vi "Module - MQTT Client.vi"(8 "error in (no error)":errorcluster) -> (0 "error in (no error) 2":errorcluster)   [LabVIEW 2020]
uses:
  <vilib>/LabVIEW Open Source Project/MQTT Connection/MQTT_Base/Base Class/MQTT_Base.lvclass
  <vilib>/LabVIEW Open Source Project/MQTT Client/Client class/Client.lvclass
  Control/State - MQTT Client.ctl
  Shared/Control/State - eFGV.ctl
  <vilib>/LabVIEW Open Source Project/MQTT TCP Connection/MQTT_TCP/Connection/TCPConnection.lvclass
  <vilib>/LabVIEW Open Source Project/MQTT Control Packets/Control Packets/CONNACK/Connect Return Code -- enum.ctl
  <vilib>/LabVIEW Open Source Project/MQTT Control Packets/Control Packets/CONNACK/CONNACK.lvclass
  <vilib>/LabVIEW Open Source Project/MQTT Control Packets/Control Packets/PUBLISH/PUBLISH.lvclass
  <vilib>/LabVIEW Open Source Project/MQTT Client/Client class/Public Events -- cluster.ctl
  Control/MQTT Sub Unsub.ctl
  Control/MQTT Connection Settings.ctl
  Control/MQTT Send Data.ctl
  Control/MQTT Received Data.ctl
  <vilib>/LabVIEW Open Source Project/OpenSerializer/Serializer/Serializer.lvclass
  Control/Config File Section List.ctl
  C:/Program Files (x86)/National Instruments/LabVIEW 2020/vi.lib/LabVIEW Open Source Project/MQTT Connection/MQTT_Base/Base Class/MQTT_Base.lvclass
  C:/Program Files (x86)/National Instruments/LabVIEW 2020/vi.lib/LabVIEW Open Source Project/MQTT Client/Client class/Client.lvclass
  C:/Program Files (x86)/National Instruments/LabVIEW 2020/vi.lib/LabVIEW Open Source Project/MQTT Connection/MQTT_Connection/Connection/Connection.lvclass
  C:/Program Files (x86)/National Instruments/LabVIEW 2020/vi.lib/LabVIEW Open Source Project/MQTT TCP Connection/MQTT_TCP/Connection/TCPConnection.lvclass
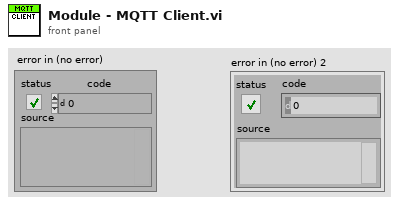
[diagram p1: front panel]
types:
  T1 = cluster{"MQTT Event":refnum<event-registration>, "eFGV Event":refnum<event-registration>}
  T2 = typedef "MQTT Send Data.ctl" = cluster{"Sender Module":string, "Receiving Module":string, "Topic":string, "Data":variant}
  T3 = typedef "MQTT Sub Unsub.ctl" = cluster{"Operation":enum16{"Subscribe", "Unsubscribe"}, "Topic Name":string[]}
  T4 = typedef "MQTT Received Data.ctl" = cluster{"Receiving Module":string, "Topic":string, "Data":variant}
  T5 = typedef "MQTT Connection Settings.ctl" = cluster{"Broker address":string, "Remote port":u16}
  T6 = cluster{"TOut":i32, "User exit":bool, "MQTT Client out":refnum<class "Client.lvclass">, "MQTT Connected":bool, "MQTT Send Data":T2, "MQTT Sub Unsub":T3, "MQTT Received Data":T4, "MQTT Connection Settings":T5, "PUBLISH":refnum<class "PUBLISH.lvclass">}
  T7 = typedef "State - MQTT Client.ctl" = enum16{"Init module", "Register event", "Idle", "Init MQTT Connections", "Init Subscribe Topic", "Create MQTT Client", "Register MQTT Event", "Connect to MQTT Server", "Subscribe MQTT Topic", "Publish to MQTT Tag", "Read MQTT Tag", "Send eFGV", "Check MQTT Connection", "Disconnect from MQTT Server", "Unregister eFGV event", "Close module"}
  T8 = typedef "Config File Section List.ctl" = enum16{"RasPi Setting", "MQTT Server Setting", "MQTT Client Setting", "WiFi Setting", "MQTT Topics"}
  T9 = typedef "State - eFGV.ctl" = enum16{"Init", "Read", "Write", "Close"}
  T10 = typedef "MQTT Client.lvlib/Client.lvclass/Public Events -- cluster.ctl" = cluster{"Connection Status":refnum<user-event>, "Connected":refnum<user-event>, "Application Message":refnum<user-event>}
  T11 = typedef "MQTT Base.lvlib/MQTT_Base.lvclass/Public Events -- cluster.ctl" = cluster{"Stop Event":refnum<user-event>, "Error Event":refnum<user-event>, "Inbound Message":refnum<user-event>}
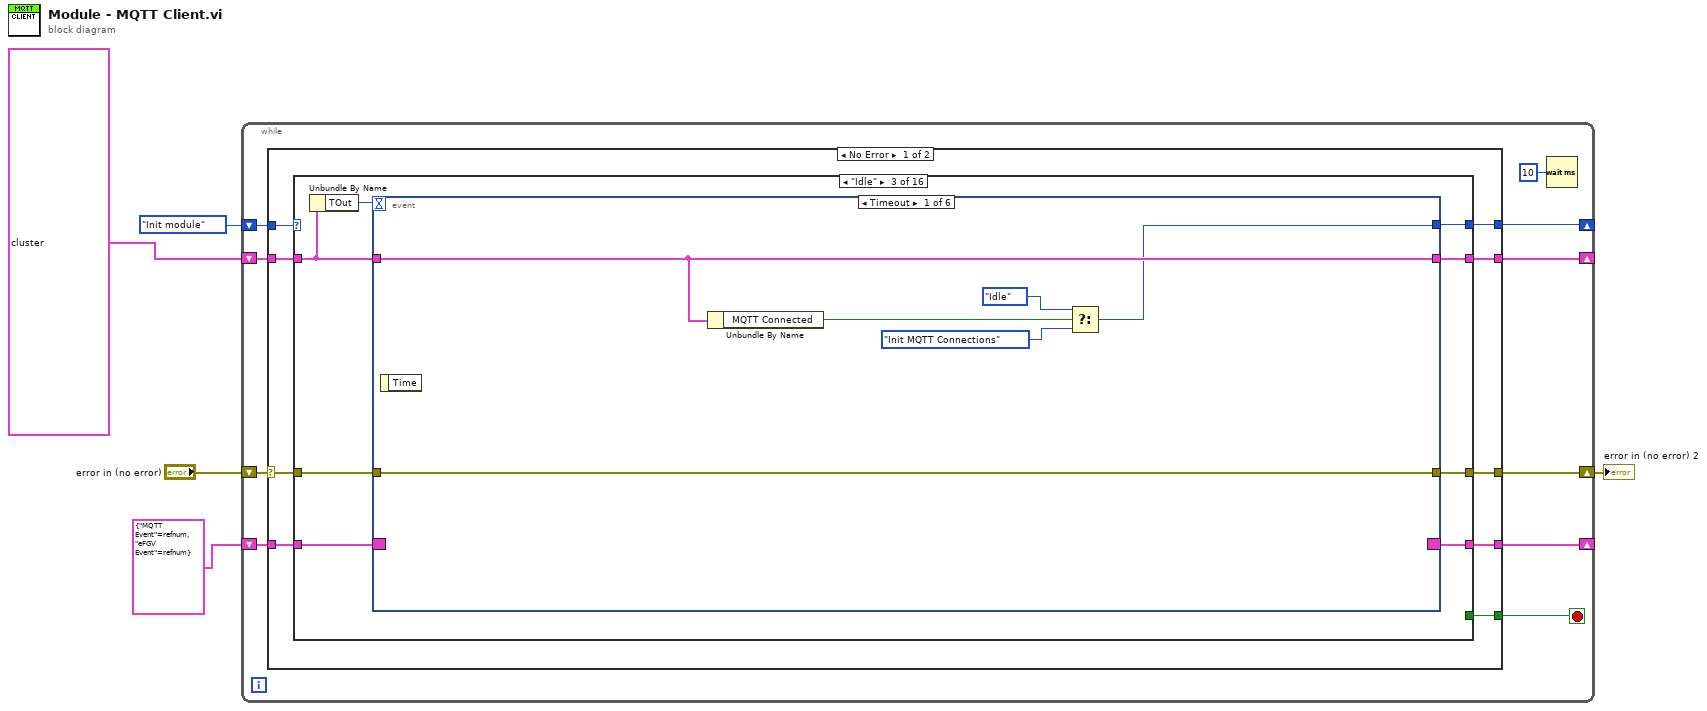
[diagram p0: block diagram]
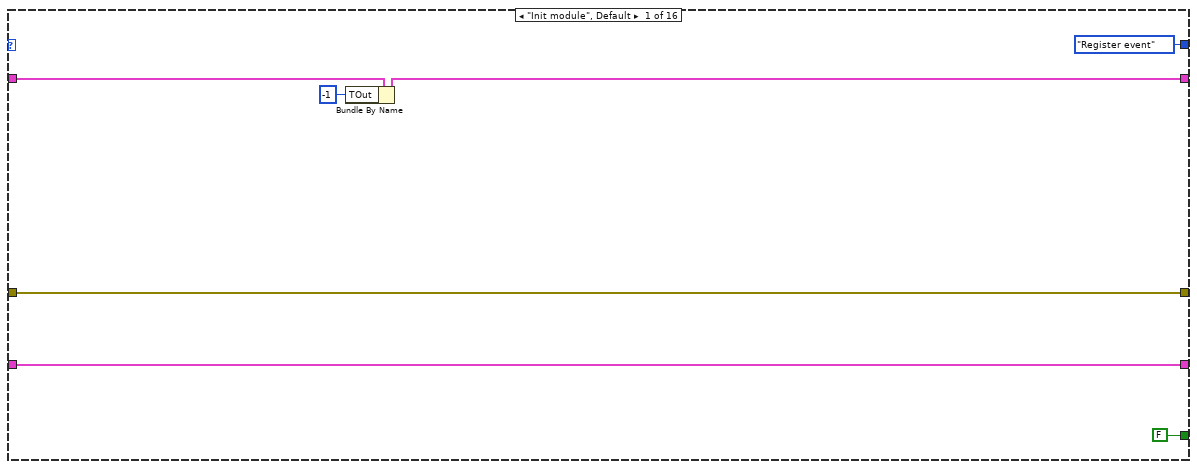
[diagram p2: hidden frame]
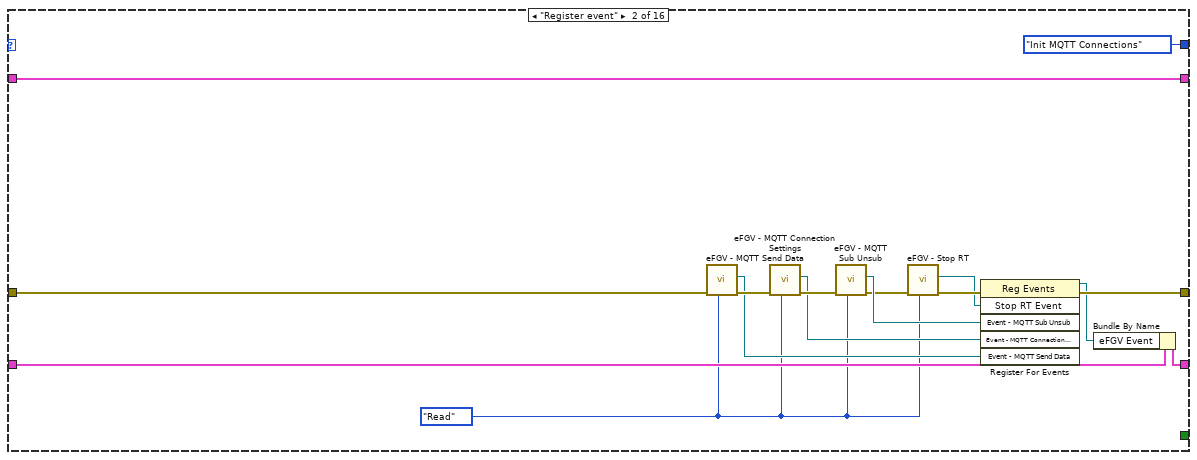
[diagram p3: hidden frame]
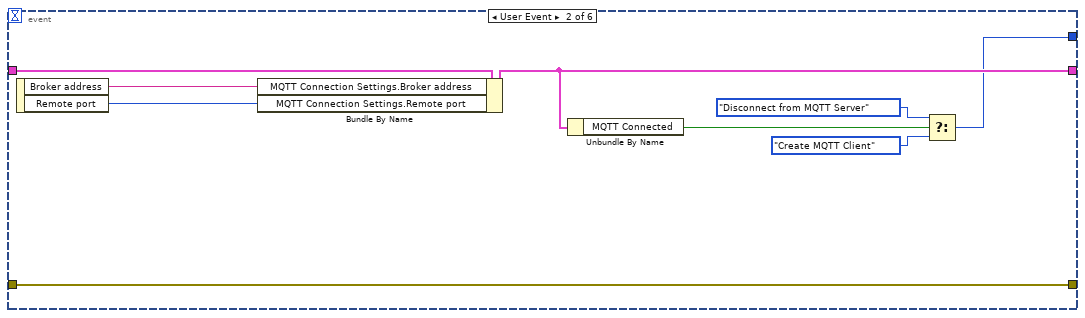
[diagram p4: hidden frame]
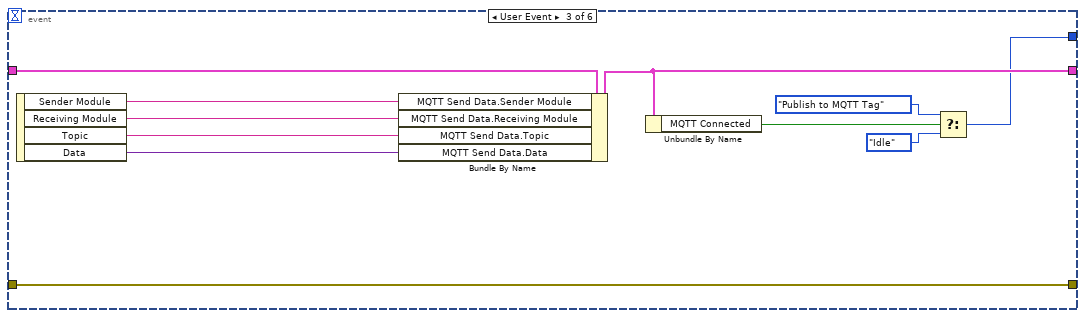
[diagram p5: hidden frame]
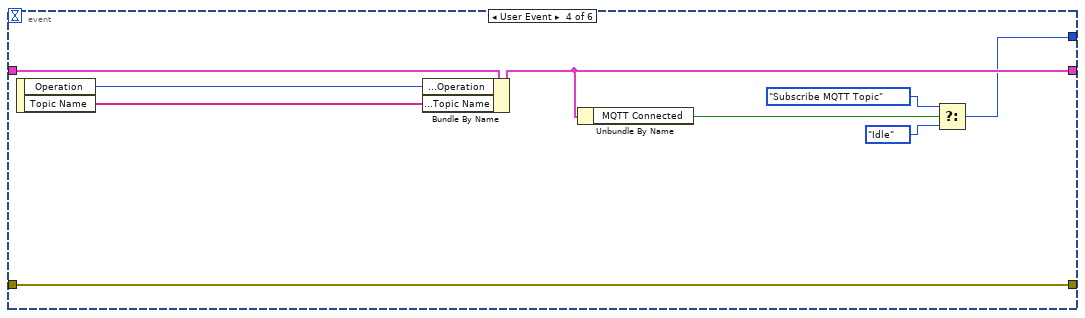
[diagram p6: hidden frame]
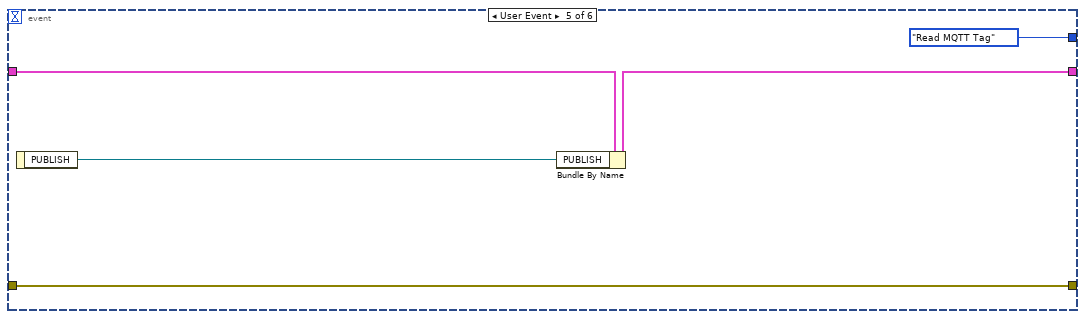
[diagram p7: hidden frame]
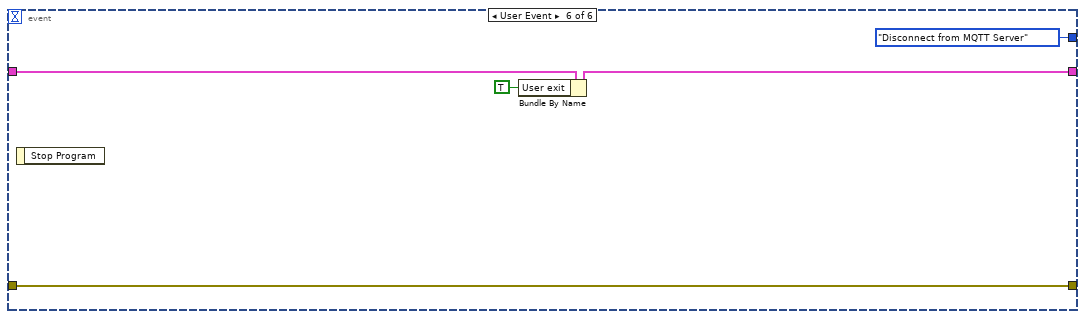
[diagram p8: hidden frame]
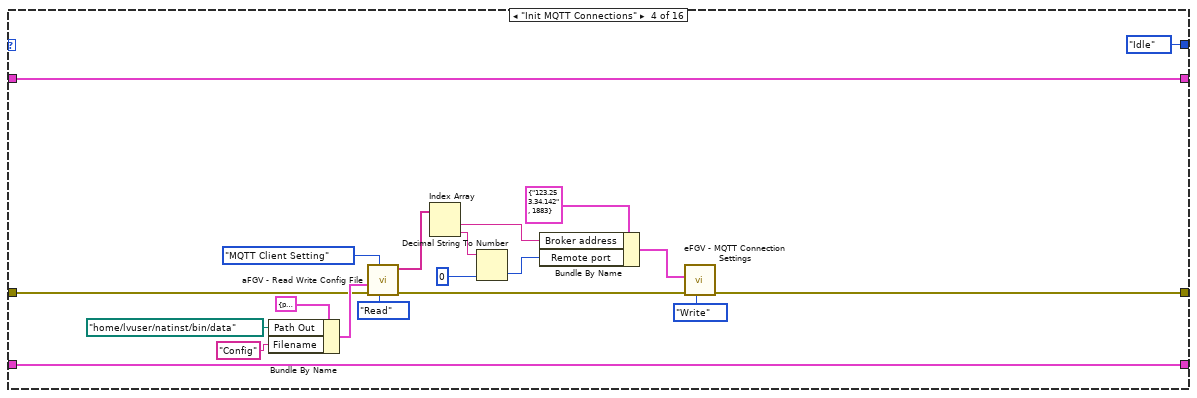
[diagram p9: hidden frame]
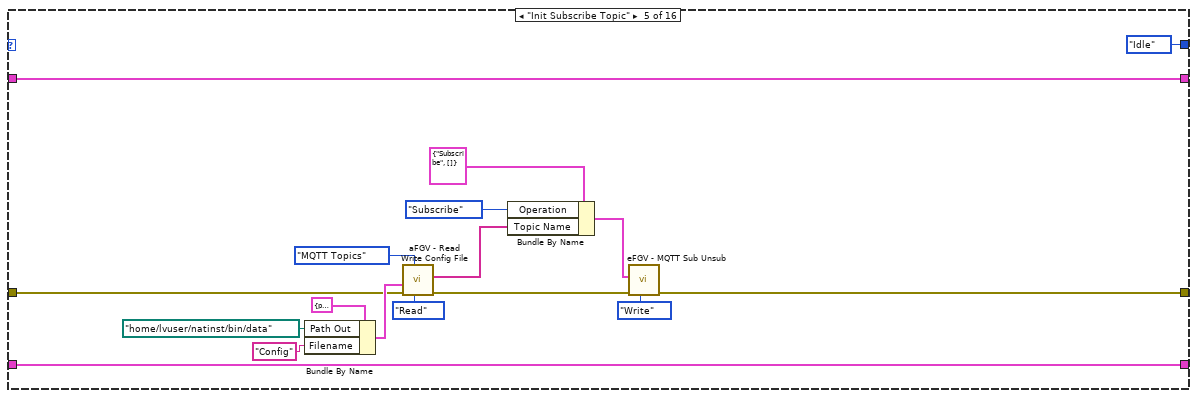
[diagram p10: hidden frame]
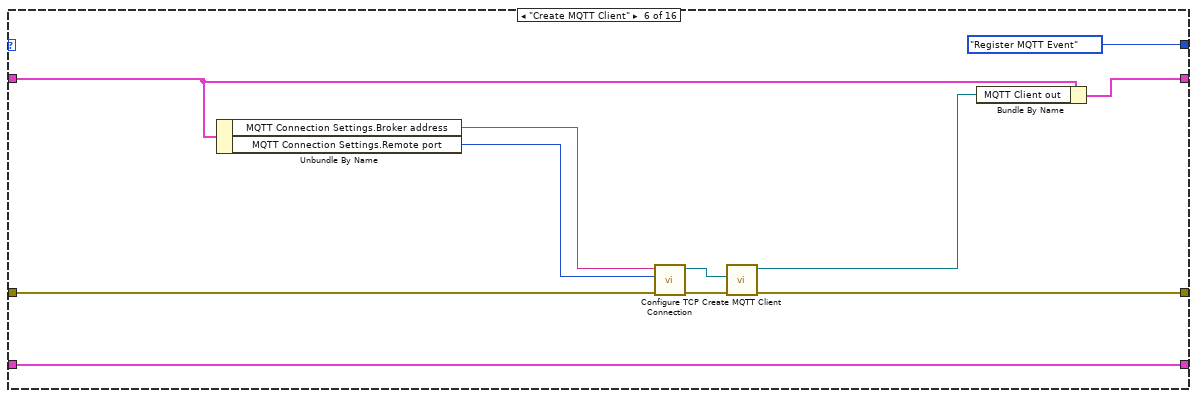
[diagram p11: hidden frame]
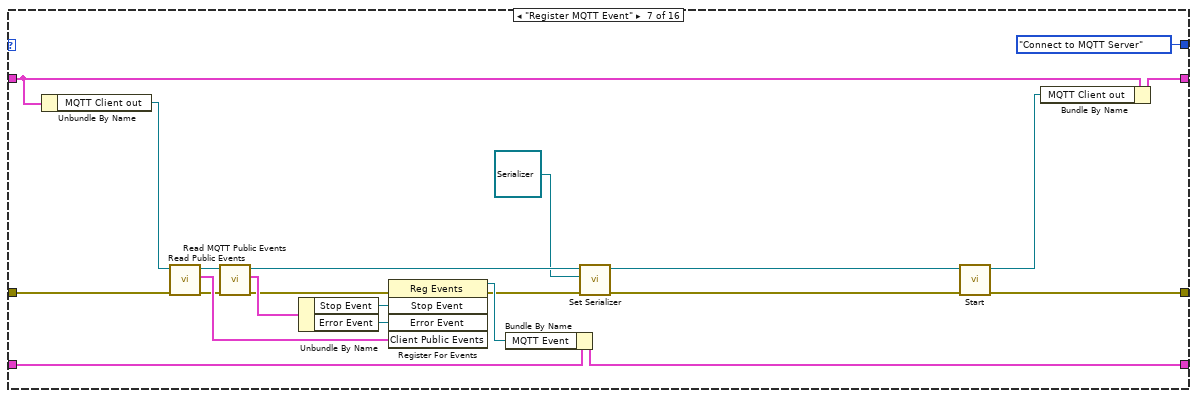
[diagram p12: hidden frame]
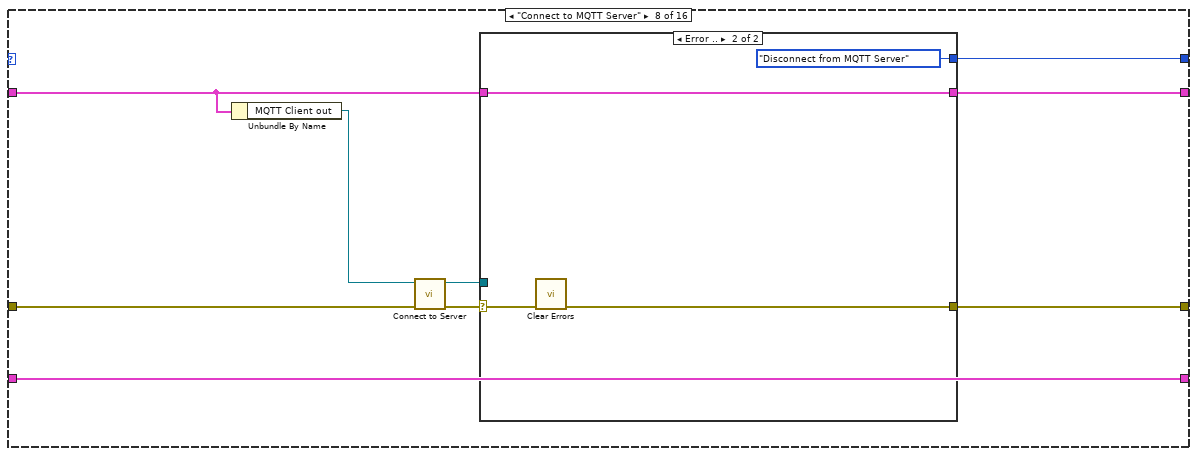
[diagram p13: hidden frame]
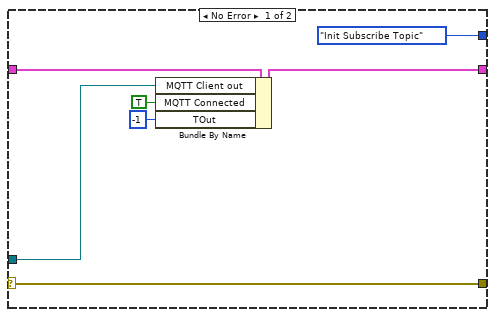
[diagram p14: hidden frame]
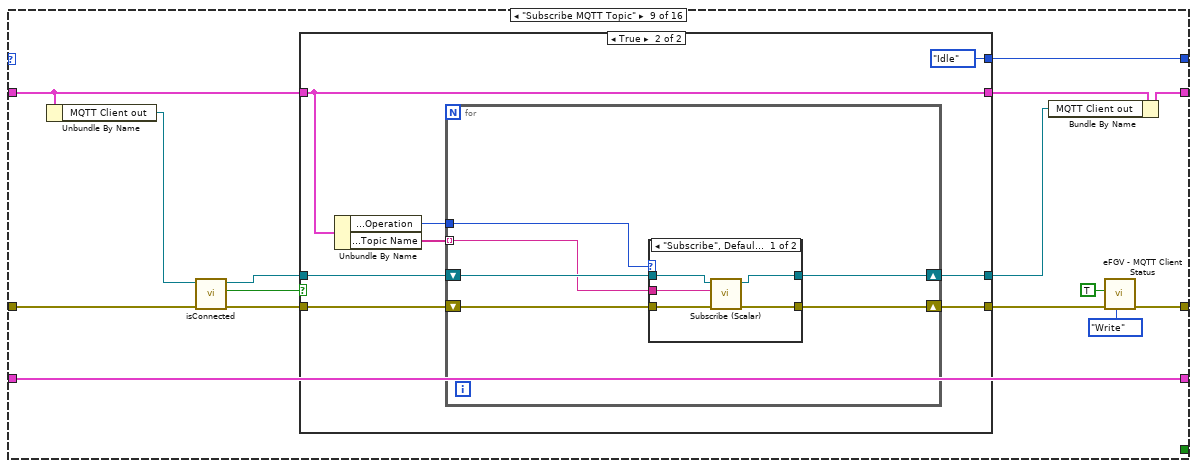
[diagram p15: hidden frame]
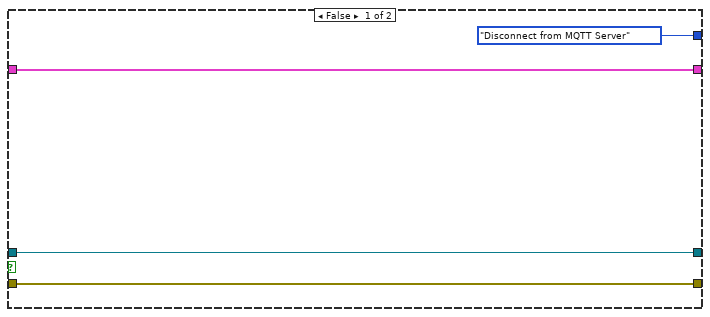
[diagram p16: hidden frame]
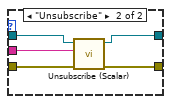
[diagram p17: hidden frame]
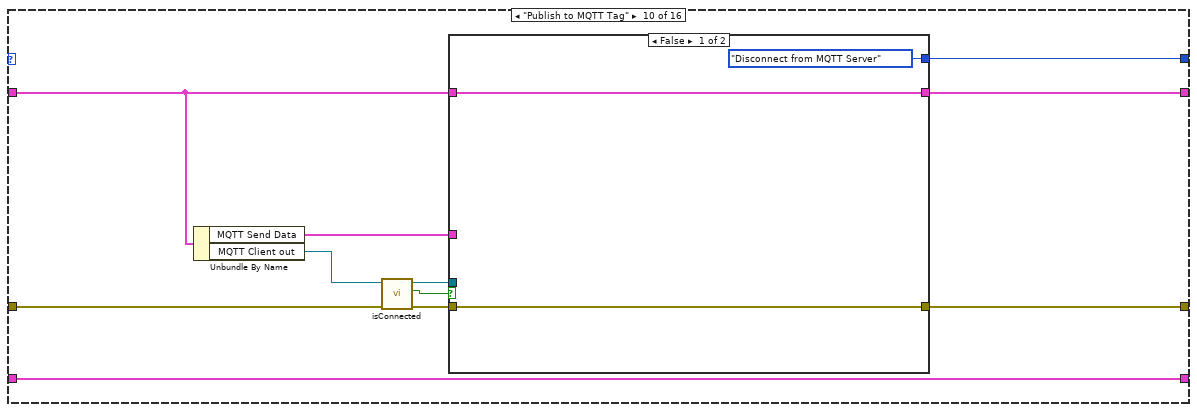
[diagram p18: hidden frame]
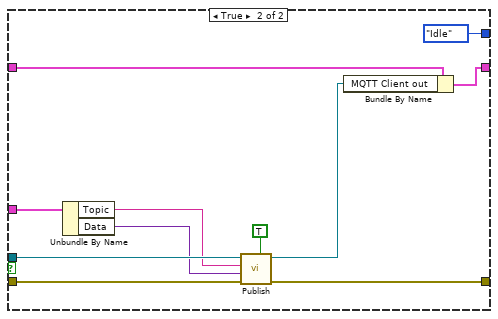
[diagram p19: hidden frame]
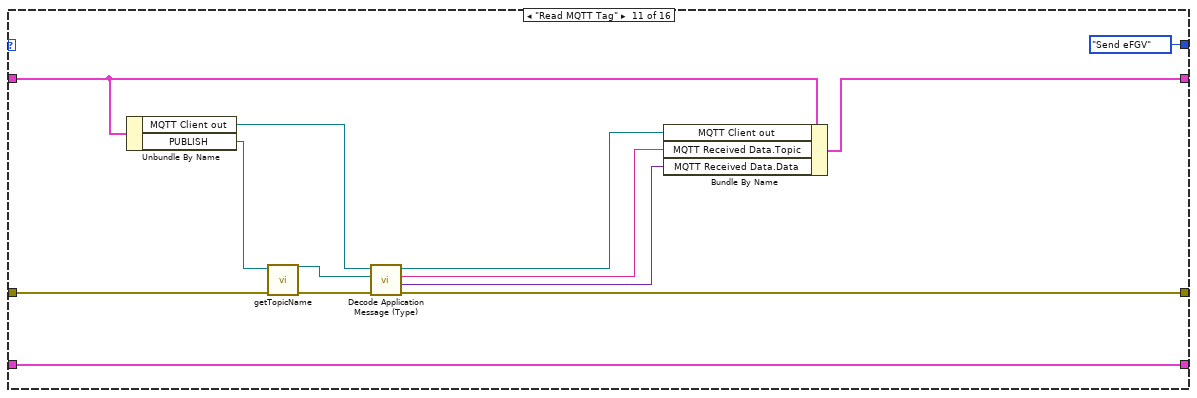
[diagram p20: hidden frame]
diagram:
  n1 = while {
    shift-right: [w12] -> _
    shift-left: State_-_MQTT_Client."Init module" -> [w15]
    shift-right: [w13] -> w1
    shift-left: "error in (no error)" -> [w14]
    shift-right: [w9] -> _
    shift-left: T6 {"TOut"=-1, "User exit"=FALSE, "MQTT Client out"=refnum, "MQTT Connected"=FALSE, "MQTT Send Data"={"Sender Module"="", "Receiving Module"="", "Topic"="", "Data"=variant}, "MQTT Sub Unsub"={"Operation"=enum."Subscribe", "Topic Name"=[]}, "MQTT Received Data"={"Receiving Module"="", "Topic"="", "Data"=variant}, "MQTT Connection Settings"={"Broker address"="123.253.34.142", "Remote port"=1883}, "PUBLISH"=refnum} -> [w10]
    shift-right: [w7] -> _
    shift-left: T1 {"MQTT Event"=refnum, "eFGV Event"=refnum} -> [w8]
    stop <- w11 stop-if-true
    n2 = case shown="No Error" w14 {
      selector: w14 -> [w23 w335]
      tunnel: w15 -> [w24 _]
      tunnel: [w22 w333] -> w13
      tunnel: [w21 State_-_MQTT_Client."Idle"] -> w12
      tunnel: [w20 _] -> w11
      tunnel: w10 -> [w19 w331]
      tunnel: [w18 w331] -> w9
      tunnel: w8 -> [w17 w330]
      tunnel: [w16 w330] -> w7
      frame No Error {
        n3 = case shown="\"Idle\"" w24 {
          tunnel: w23 -> [w31 w38 w49 w107 w125 w145 w162 w178 w204 w242 w265 w277 w284 w302 w321 w329]
          tunnel: [w31 w45 w48 w118 w135 w143 w161 w172 w191 w243 w264 w276 w283 w287 w320 w329] -> w22
          tunnel: [State_-_MQTT_Client."Register event" State_-_MQTT_Client."Init MQTT Connections" w52 State_-_MQTT_Client."Idle" State_-_MQTT_Client."Idle" State_-_MQTT_Client."Register MQTT Event" State_-_MQTT_Client."Connect to MQTT Server" w171 w195 w234 State_-_MQTT_Client."Send eFGV" State_-_MQTT_Client."Idle" _ w293 State_-_MQTT_Client."Close module" State_-_MQTT_Client."Close module"] -> w21
          tunnel: [FALSE _ _ _ _ _ _ _ _ _ _ _ _ _ _ TRUE] -> w20
          tunnel: w19 -> [w28 w47 w51 w120 w137 w140 w158 w177 w200 w236 w262 w278 w282 w295 w324 w328]
          tunnel: [w26 w47 w50 w120 w137 w141 w160 w175 w197 w235 w263 w278 w282 w292 w324 w328] -> w18
          tunnel: w17 -> [w27 w44 w55 w119 w136 w148 w170 w179 w205 w244 w271 w280 w285 w299 w322 w327]
          tunnel: [w27 w43 w54 w119 w136 w148 w156 w179 w205 w244 w271 w280 w285 w298 w322 w327] -> w16
          frame "Init module", Default {
            n4 = Bundle By Name(cluster=w28, "TOut"=-1) -> (w26:T6)
          }
          frame "Register event" {
            w32 = State_-_eFGV."Read" ("State")
            n5 = call "eFGV - MQTT Send Data.vi"("State"=w32, "error in (no error)"=w38) -> ("error out"=w37:errorcluster, "Event - MQTT Send Data"=w36:refnum<user-event>)  [unwired: 8 in]
            n6 = call "eFGV - MQTT Connection Settings.vi"("State"=w32, "error in (no error)"=w37) -> ("error out"=w40:errorcluster, "Event - MQTT Connection Settings"=w39:refnum<user-event>)  [unwired: 8 in]
            n7 = call "eFGV - MQTT Sub Unsub.vi"("State"=w32, "error in (no error)"=w40) -> ("error out"=w35:errorcluster, "Event - MQTT Sub Unsub"=w42:refnum<user-event>)  [unwired: 8 in]
            n8 = call "eFGV - Stop RT.vi"("State"=w32, "error in (no error)"=w35) -> ("error out"=w34:errorcluster, "Stop RT Event"=w33:refnum<user-event>)  [unwired: 8 in]
            n9 = register-events(error in=w34, w33, w42, w39, w36) -> (reference out=w41:refnum<event-registration>, error out=w45:errorcluster)  [unwired: 1 in]
            n10 = Bundle By Name(cluster=w44, "eFGV Event"=w41) -> (w43:T1)
          }
          frame "Idle" {
            n11 = Unbundle By Name(w51) -> ("TOut"=w53:i32)
            n12 = event shown="[0] Timeout" {
              selector: w55 -> [_ _ _ _ _ _]
              dyn-events: [_ _ _ _ _ _] -> w54
              timeout: w53 -> [_ _ _ _ _ _]
              tunnel: [w56 w62 w73 w82 State_-_MQTT_Client."Read MQTT Tag" State_-_MQTT_Client."Disconnect from MQTT Server"] -> w52
              tunnel: w51 -> [w60 w70 w81 w90 w94 w99]
              tunnel: [w60 w63 w74 w86 w93 w98] -> w50
              tunnel: w49 -> [w61 w67 w78 w89 w95 w96]
              tunnel: [w61 w67 w78 w89 w95 w96] -> w48
              event Timeout {
                n13 = event-data() -> ()  [unwired: 1 in, 1 out]
                n14 = Unbundle By Name(w60) -> ("MQTT Connected"=w59:bool)
                n15 = Select(t=State_-_MQTT_Client."Idle", s=w59, f=State_-_MQTT_Client."Init MQTT Connections") -> (s? t:f=w56:T7)
              }
              event User Event {
                n16 = event-data() -> ("Broker address"=w69:string, "Remote port"=w68:u16)  [unwired: 1 in]
                n17 = Bundle By Name(cluster=w70, "MQTT Connection Settings.Broker address"=w69, "MQTT Connection Settings.Remote port"=w68) -> (w63:T6)
                n18 = Unbundle By Name(w63) -> ("MQTT Connected"=w66:bool)
                n19 = Select(t=State_-_MQTT_Client."Disconnect from MQTT Server", s=w66, f=State_-_MQTT_Client."Create MQTT Client") -> (s? t:f=w62:T7)
              }
              event User Event {
                n20 = event-data() -> ("Sender Module"=w72:string, "Receiving Module"=w71:string, "Topic"=w79:string, "Data"=w80:variant)  [unwired: 1 in]
                n21 = Bundle By Name(cluster=w81, "MQTT Send Data.Sender Module"=w72, "MQTT Send Data.Receiving Module"=w71, "MQTT Send Data.Topic"=w79, "MQTT Send Data.Data"=w80) -> (w74:T6)
                n22 = Unbundle By Name(w74) -> ("MQTT Connected"=w77:bool)
                n23 = Select(t=State_-_MQTT_Client."Publish to MQTT Tag", s=w77, f=State_-_MQTT_Client."Idle") -> (s? t:f=w73:T7)
              }
              event User Event {
                n24 = event-data() -> ("Operation"=w87:enum16{"Subscribe", "Unsubscribe"}, "Topic Name"=w88:string[])  [unwired: 1 in]
                n25 = Bundle By Name(cluster=w90, "MQTT Sub Unsub.Operation"=w87, "MQTT Sub Unsub.Topic Name"=w88) -> (w86:T6)
                n26 = Unbundle By Name(w86) -> ("MQTT Connected"=w85:bool)
                n27 = Select(t=State_-_MQTT_Client."Subscribe MQTT Topic", s=w85, f=State_-_MQTT_Client."Idle") -> (s? t:f=w82:T7)
              }
              event User Event {
                n28 = event-data() -> ("PUBLISH"=w91:refnum<class "PUBLISH.lvclass">)  [unwired: 1 in]
                n29 = Bundle By Name(cluster=w94, "PUBLISH"=w91) -> (w93:T6)
              }
              event User Event {
                n30 = event-data() -> ()  [unwired: 1 in, 1 out]
                n31 = Bundle By Name(cluster=w99, "User exit"=TRUE) -> (w98:T6)
              }
            }
          }
          frame "Init MQTT Connections" {
            n32 = Bundle By Name(cluster=cluster{"Path Out":path, "Filename":string} {"Path Out"=path "", "Filename"=""} ("Path File"), "Path Out"=path "/home/lvuser/natinst/bin/data", "Filename"="Config") -> (w108:cluster{"Path Out":path, "Filename":string})
            n33 = call "aFGV - Read Write Config File.vi"("State"=enum16{"Read", "Write", "Delete"}."Read", "Section"=Config_File_Section_List."MQTT Client Setting", "Error In"=w107, "Path File"=w108) -> ("Error Out"=w106:errorcluster, "Data out"=w105:string[])  [unwired: 5 in, 1 out]
            n34 = Index Array(array=w105) -> (element #1=w104:string, element #2=w103:string)  [unwired: 2 in]
            n35 = Decimal String To Number(string=w103, default (0L)=u16 0 ("Remote port")) -> (number=w101:u16)  [unwired: 1 in, 1 out]
            n36 = Bundle By Name(cluster=T5 {"Broker address"="123.253.34.142", "Remote port"=1883} ("MQTT Connection Settings"), "Broker address"=w104, "Remote port"=w101) -> (w116:T5)
            n37 = call "eFGV - MQTT Connection Settings.vi"("State"=State_-_eFGV."Write", "error in (no error)"=w106, "MQTT Connection Settings"=w116) -> ("error out"=w118:errorcluster)  [unwired: 7 in, 1 out]
          }
          frame "Init Subscribe Topic" {
            n38 = Bundle By Name(cluster=cluster{"Path Out":path, "Filename":string} {"Path Out"=path "", "Filename"=""} ("Path File"), "Path Out"=path "/home/lvuser/natinst/bin/data", "Filename"="Config") -> (w127:cluster{"Path Out":path, "Filename":string})
            n39 = call "aFGV - Read Write Config File.vi"("State"=enum16{"Read", "Write", "Delete"}."Read", "Section"=Config_File_Section_List."MQTT Topics", "Error In"=w125, "Path File"=w127) -> ("Error Out"=w126:errorcluster, "Key Names Out"=w122:string[])  [unwired: 5 in, 1 out]
            n40 = Bundle By Name(cluster=T3 {"Operation"=enum."Subscribe", "Topic Name"=[]} ("MQTT Sub Unsub"), "Operation"=enum16{"Subscribe", "Unsubscribe"}."Subscribe", "Topic Name"=w122) -> (w121:T3)
            n41 = call "eFGV - MQTT Sub Unsub.vi"("State"=State_-_eFGV."Write", "error in (no error)"=w126, "MQTT Sub Unsub"=w121) -> ("error out"=w135:errorcluster)  [unwired: 7 in, 1 out]
          }
          frame "Create MQTT Client" {
            n42 = Unbundle By Name(w140) -> ("MQTT Connection Settings.Broker address"=w139:string, "MQTT Connection Settings.Remote port"=w138:u16)
            n43 = call <vilib>:"Configure TCP Connection.vi"("error in (no error)"=w145, "remote port (80)"=w138, "address (localhost)"=w139) -> ("error out"=w146:errorcluster, "TCPConnection"=w147:refnum<class "TCPConnection.lvclass">)  [unwired: 7 in]
            n44 = call <vilib>:"Create MQTT Client.vi"("error in (no error)"=w146, "Connection Configuration"=w147) -> ("error out"=w143:errorcluster, "Client out"=w142:refnum<class "Client.lvclass">)  [unwired: 8 in]
            n45 = Bundle By Name(cluster=w140, "MQTT Client out"=w142) -> (w141:T6)
          }
          frame "Register MQTT Event" {
            n46 = Unbundle By Name(w158) -> ("MQTT Client out"=w157:refnum<class "Client.lvclass">)
            n47 = call <vilib>:"Read Public Events.vi"("error in (no error)"=w162, "Client in"=w157) -> ("error out"=w164:errorcluster, "Client Public Events"=w166:T10, "Client out"=w163:refnum<class "Client.lvclass">)  [unwired: 7 in]
            n48 = call <vilib>:"Read MQTT Public Events.vi"("error in (no error)"=w164, "MQTT_Base in"=w163) -> ("error out"=w165:errorcluster, "MQTT Public Events"=w169:T11, "MQTT_Base out"=w151:refnum<class "Client.lvclass">)  [unwired: 7 in]
            n49 = Unbundle By Name(w169) -> ("Stop Event"=w167:refnum<user-event>, "Error Event"=w168:refnum<user-event>)
            n50 = register-events(error in=w165, w167, w168, w166) -> (reference out=w155:refnum<event-registration>, error out=w153:errorcluster)  [unwired: 1 in]
            n51 = Bundle By Name(cluster=w170, "MQTT Event"=w155) -> (w156:T1)
            n52 = call <vilib>:"Set Serializer.vi"("error in (no error)"=w153, "Serializer (default: Flattened String)"=refnum<class "Serializer.lvclass"> refnum, "MQTT_Base"=w151) -> ("error out"=w152:errorcluster, "MQTT_Base out"=w150:refnum<class "Client.lvclass">)  [unwired: 7 in]
            n53 = call <vilib>:"Start.vi"("error in (no error)"=w152, "MQTT_Base in"=w150) -> ("error out"=w161:errorcluster, "MQTT_Base out"=w159:refnum<class "Client.lvclass">)  [unwired: 7 in, 1 out]
            n54 = Bundle By Name(cluster=w158, "MQTT Client out"=w159) -> (w160:T6)
          }
          frame "Connect to MQTT Server" {
            n55 = Unbundle By Name(w177) -> ("MQTT Client out"=w176:refnum<class "Client.lvclass">)
            n56 = call <vilib>:"Connect to Server.vi"("error in (no error)"=w178, "Client in"=w176) -> ("error out"=w173:errorcluster, "Client out"=w174:refnum<class "Client.lvclass">)  [unwired: 6 in, 2 out]
            n57 = case shown="Error .." w173 {
              selector: w173 -> [w182 w189]
              tunnel: w177 -> [w186 w190]
              tunnel: [w185 w190] -> w175
              tunnel: w174 -> [w184 _]
              tunnel: [w182 w188] -> w172
              tunnel: [State_-_MQTT_Client."Init Subscribe Topic" State_-_MQTT_Client."Disconnect from MQTT Server"] -> w171
              frame No Error {
                n58 = Bundle By Name(cluster=w186, "MQTT Client out"=w184, "MQTT Connected"=TRUE, "TOut"=-1) -> (w185:T6)
              }
              frame Error {
                n59 = call <vilib>:"Clear Errors.vi"("error in (no error)"=w189) -> ("error out"=w188:errorcluster)  [unwired: 5 in, 1 out]
              }
            }
          }
          frame "Subscribe MQTT Topic" {
            n60 = Unbundle By Name(w200) -> ("MQTT Client out"=w201:refnum<class "Client.lvclass">)
            n61 = call <vilib>:"isConnected.vi"("error in (no error)"=w204, "Client in"=w201) -> ("error out"=w202:errorcluster, "connected"=w203:bool, "Client out"=w199:refnum<class "Client.lvclass">)  [unwired: 7 in]
            n62 = case shown="True" w203 {
              tunnel: w202 -> [w209 w214]
              tunnel: w200 -> [w207 w217]
              tunnel: w199 -> [w208 w212]
              tunnel: [w207 w217] -> w198
              tunnel: [w209 w213] -> w192
              tunnel: [w208 w211] -> w196
              tunnel: [State_-_MQTT_Client."Disconnect from MQTT Server" State_-_MQTT_Client."Idle"] -> w195
              frame False {
              }
              frame True {
                n63 = Unbundle By Name(w217) -> ("MQTT Sub Unsub.Operation"=w215:enum16{"Subscribe", "Unsubscribe"}, "MQTT Sub Unsub.Topic Name"=w216:string[])
                n64 = for {
                  tunnel: w216 -> [w220] mode=indexing
                  tunnel: w215 -> [w219]
                  shift-right: [w218] -> w211
                  shift-left: w212 -> [w221]
                  shift-right: [w222] -> w213
                  shift-left: w214 -> [w223]
                  n65 = case shown="\"Subscribe\", Default" w219 {
                    tunnel: w223 -> [w228 w233]
                    tunnel: [w227 w232] -> w222
                    tunnel: w221 -> [w226 w230]
                    tunnel: w220 -> [w225 w231]
                    tunnel: [w224 w229] -> w218
                    frame "Subscribe", Default {
                      n66 = call <vilib>:"Subscribe (Scalar).vi"("error in (no error)"=w228, "Topic Filter"=w225, "Client in"=w226) -> ("error out"=w227:errorcluster, "Client out"=w224:refnum<class "Client.lvclass">)  [unwired: 6 in, 1 out]
                    }
                    frame "Unsubscribe" {
                      n67 = call <vilib>:"Unsubscribe (Scalar).vi"("error in (no error)"=w233, "Topic Filter"=w231, "Client in"=w230) -> ("error out"=w232:errorcluster, "Client out"=w229:refnum<class "Client.lvclass">)  [unwired: 6 in, 1 out]
                    }
                  }
                }
              }
            }
            n68 = Bundle By Name(cluster=w198, "MQTT Client out"=w196) -> (w197:T6)
            n69 = call "eFGV - MQTT Client Status.vi"("State"=State_-_eFGV."Write", "error in (no error)"=w192, "MQTT Connected"=TRUE) -> ("error out"=w191:errorcluster)  [unwired: 7 in, 1 out]
          }
          frame "Publish to MQTT Tag" {
            n70 = Unbundle By Name(w236) -> ("MQTT Send Data"=w237:T2, "MQTT Client out"=w240:refnum<class "Client.lvclass">)
            n71 = call <vilib>:"isConnected.vi"("error in (no error)"=w242, "Client in"=w240) -> ("error out"=w241:errorcluster, "connected"=w238:bool, "Client out"=w239:refnum<class "Client.lvclass">)  [unwired: 7 in]
            n72 = case shown="False" w238 {
              tunnel: [w247 w258] -> w243
              tunnel: w241 -> [w247 w257]
              tunnel: w239 -> [_ w256]
              tunnel: w237 -> [_ w255]
              tunnel: w236 -> [w245 w252]
              tunnel: [w245 w251] -> w235
              tunnel: [State_-_MQTT_Client."Disconnect from MQTT Server" State_-_MQTT_Client."Idle"] -> w234
              frame False {
              }
              frame True {
                n73 = Unbundle By Name(w255) -> ("Topic"=w254:string, "Data"=w253:variant)
                n74 = call <vilib>:"Publish.vi"("RETAIN"=TRUE, "error in (no error)"=w257, "Payload"=w253, "Topic Name (empty: Payload name)"=w254, "Client in"=w256) -> ("error out"=w258:errorcluster, "Client out"=w250:refnum<class "Client.lvclass">)  [unwired: 4 in, 1 out]
                n75 = Bundle By Name(cluster=w252, "MQTT Client out"=w250) -> (w251:T6)
              }
            }
          }
          frame "Read MQTT Tag" {
            n76 = Unbundle By Name(w262) -> ("MQTT Client out"=w259:refnum<class "Client.lvclass">, "PUBLISH"=w261:refnum<class "PUBLISH.lvclass">)
            n77 = call <vilib>:"getTopicName.vi"("error in (no error)"=w265, "PUBLISH in"=w261) -> ("error out"=w266:errorcluster, "PUBLISH out"=w267:refnum<class "PUBLISH.lvclass">)  [unwired: 7 in, 1 out]
            n78 = call <vilib>:"Decode Application Message (Type).vi"("error in (no error)"=w266, "PUBLISH"=w267, "Client in"=w259) -> ("error out"=w264:errorcluster, "Payload"=w260:variant, "Topic"=w268:string, "Client out"=w269:refnum<class "Client.lvclass">)  [unwired: 5 in]
            n79 = Bundle By Name(cluster=w262, "MQTT Client out"=w269, "MQTT Received Data.Topic"=w268, "MQTT Received Data.Data"=w260) -> (w263:T6)
          }
          frame "Send eFGV" {
            n80 = Unbundle By Name(w278) -> ("MQTT Received Data"=w274:T4, "MQTT Send Data.Receiving Module"=w273:string)
            n81 = Bundle By Name(cluster=w274, "Receiving Module"=w273) -> (w272:T4)
            n82 = call "eFGV - MQTT Received Data.vi"("State"=State_-_eFGV."Write", "error in (no error)"=w277, "MQTT Received Data"=w272) -> ("error out"=w276:errorcluster)  [unwired: 7 in, 1 out]
          }
          frame "Check MQTT Connection" {
            # "Write to Connection eFGV"
            n83 = Unbundle By Name(w282) -> ("MQTT Client out"=w281:refnum<class "Client.lvclass">)
            n84 = call <vilib>:"isConnected.vi"("error in (no error)"=w284, "Client in"=w281) -> ("error out"=w283:errorcluster)  [unwired: 7 in, 2 out]
          }
          frame "Disconnect from MQTT Server" {
            n85 = Unbundle By Name(w295) -> ("MQTT Connected"=w301:bool, "MQTT Client out"=w300:refnum<class "Client.lvclass">)
            n86 = case shown="True" w301 {
              tunnel: w302 -> [w304 w318]
              tunnel: [w304 w305] -> w288
              tunnel: w300 -> [_ w315]
              tunnel: w299 -> [w303 w310]
              tunnel: [w303 w310] -> w298
              frame False {
              }
              frame True {
                n87 = call <vilib>:"Disconnect from Server.vi"("error in (no error)"=w318, "Client in"=w315) -> ("error out"=w317:errorcluster, "Client out"=w316:refnum<class "Client.lvclass">)  [unwired: 7 in, 1 out]
                n88 = call <vilib>:"Clear Errors.vi"("error in (no error)"=w317) -> ("error out"=w308:errorcluster)  [unwired: 5 in, 1 out]
                n89 = Unbundle By Name(w310) -> ("MQTT Event"=w309:refnum<event-registration>)
                n90 = call <vilib>:"Stop.vi"("error in (no error)"=w308, "MQTT_Base in"=w316) -> ("error out"=w314:errorcluster, "MQTT_Base out"=w311:refnum<class "Client.lvclass">)  [unwired: 7 in, 1 out]
                n91 = call <vilib>:"Clear Errors.vi"("error in (no error)"=w314) -> ("error out"=w307:errorcluster)  [unwired: 5 in, 1 out]
                n92 = Unregister For Events(event registration refnum=w309, error in=w307) -> (error out=w313:errorcluster)
                n93 = call <vilib>:"Clear Errors.vi"("error in (no error)"=w313) -> ("error out"=w306:errorcluster)  [unwired: 5 in, 1 out]
                n94 = call <vilib>:"Destroy.vi"("error in (no error)"=w306, "MQTT_Base in"=w311) -> ("error out"=w312:errorcluster)  [unwired: 8 in, 1 out]
                n95 = call <vilib>:"Clear Errors.vi"("error in (no error)"=w312) -> ("error out"=w305:errorcluster)  [unwired: 5 in, 1 out]
              }
            }
            n96 = Unbundle By Name(w295) -> ("User exit"=w294:bool)
            n97 = Select(t=State_-_MQTT_Client."Unregister eFGV event", s=w294, f=State_-_MQTT_Client."Init MQTT Connections") -> (s? t:f=w293:T7)
            n98 = Bundle By Name(cluster=w295, "MQTT Connected"=FALSE, "TOut"=100) -> (w292:T6)
            n99 = call "eFGV - MQTT Client Status.vi"("State"=State_-_eFGV."Write", "error in (no error)"=w288, "MQTT Connected"=FALSE) -> ("error out"=w287:errorcluster)  [unwired: 7 in, 1 out]
          }
          frame "Unregister eFGV event" {
            n100 = Unbundle By Name(w322) -> ("eFGV Event"=w319:refnum<event-registration>)
            n101 = Unregister For Events(event registration refnum=w319, error in=w321) -> (error out=w320:errorcluster)
          }
          frame "Close module" {
          }
        }
      }
      frame Error {
        n102 = call <vilib>:"Simple Error Handler.vi"("error in (no error)"=w335) -> ("error out"=w334:errorcluster)  [unwired: 4 in, 4 out]
        n103 = call <vilib>:"Clear Errors.vi"("error in (no error)"=w334) -> ("error out"=w333:errorcluster)  [unwired: 5 in, 1 out]
      }
    }
    n104 = Wait (ms)(milliseconds to wait=u32 10) -> ()  [unwired: 1 out]
  }
  "error in (no error) 2" <- w1
